vi "Interpreter.vi"(0 "string":string) -> (7 "RwZ":sgl[](array[numeric]), 8 "Yaw":sgl[](array[numeric]), 9 "RwY":sgl[](array[numeric]), 10 "Pitch":sgl[](array[numeric]), 11 "RwX":sgl[](array[numeric]), 12 "GyroX":sgl[](array[numeric]), 13 "AccZ":sgl[](array[numeric]), 14 "Roll":sgl[](array[numeric]), 15 "GyroY":sgl[](array[numeric]), 16 "Acc X":sgl[](array[numeric]), 17 "GyroZ":sgl[](array[numeric]), 18 "AccY":sgl[](array[numeric]))   [LabVIEW 2020]
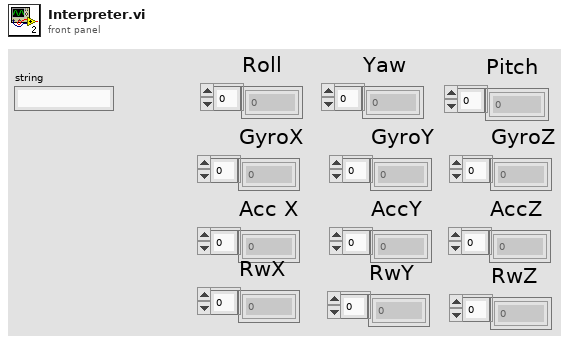
[diagram p1: front panel]
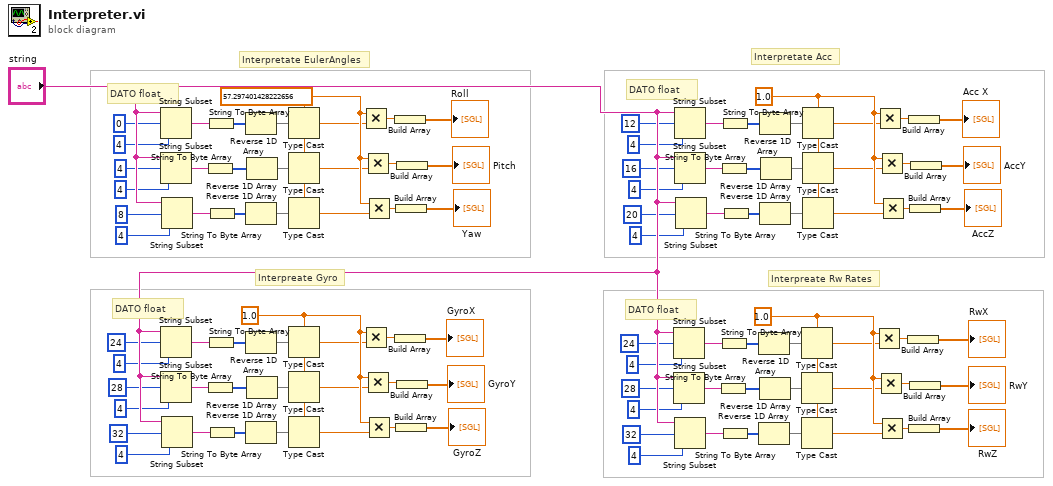
[diagram p0: block diagram]
diagram:
  w91 = sgl 1.0
  w69 = sgl 1.0
  w47 = sgl 1.0
  w22 = sgl 57.2974
  # "Interpreate Rw Rates"
  # "DATO float"
  # "Interpreate Gyro"
  # "Interpretate Acc"
  # "Interpretate EulerAngles"
  # "DATO float"
  # "DATO float"
  # "DATO float"
  n1 = String Subset(string="string", offset (0)=0, length (rest)=4 ("length (rest)")) -> (substring=w7:string)
  n2 = String Subset(string="string", offset (0)=4, length (rest)=4 ("length (rest)")) -> (substring=w8:string)
  n3 = String Subset(string="string", offset (0)=24, length (rest)=4 ("length (rest)")) -> (substring=w54:string)
  n4 = String Subset(string="string", offset (0)=28, length (rest)=4 ("length (rest)")) -> (substring=w55:string)
  n5 = String Subset(string="string", offset (0)=8, length (rest)=4 ("length (rest)")) -> (substring=w9:string)
  n6 = String Subset(string="string", offset (0)=32, length (rest)=4 ("length (rest)")) -> (substring=w56:string)
  n7 = String To Byte Array(string=w8) -> (unsigned byte array=w14:u8[])
  n8 = String To Byte Array(string=w55) -> (unsigned byte array=w61:u8[])
  n9 = String To Byte Array(string=w7) -> (unsigned byte array=w10:u8[])
  n10 = String To Byte Array(string=w54) -> (unsigned byte array=w57:u8[])
  n11 = String To Byte Array(string=w9) -> (unsigned byte array=w15:u8[])
  n12 = String To Byte Array(string=w56) -> (unsigned byte array=w62:u8[])
  n13 = Reverse 1D Array(array=w10) -> (reversed array=w11:u8[])
  n14 = Reverse 1D Array(array=w15) -> (reversed array=w13:u8[])
  n15 = Reverse 1D Array(array=w57) -> (reversed array=w58:u8[])
  n16 = Reverse 1D Array(array=w62) -> (reversed array=w60:u8[])
  n17 = Reverse 1D Array(array=w14) -> (reversed array=w12:u8[])
  n18 = Reverse 1D Array(array=w61) -> (reversed array=w59:u8[])
  n19 = Type Cast(type=w22, x=w11) -> (*(type *) &x=w17:sgl)
  n20 = Type Cast(type=w22, x=w12) -> (*(type *) &x=w18:sgl)
  n21 = Type Cast(type=w22, x=w13) -> (*(type *) &x=w19:sgl)
  n22 = Type Cast(type=w69, x=w58) -> (*(type *) &x=w64:sgl)
  n23 = Type Cast(type=w69, x=w59) -> (*(type *) &x=w65:sgl)
  n24 = Type Cast(type=w69, x=w60) -> (*(type *) &x=w66:sgl)
  n25 = Multiply(x=w22, y=w17) -> (x*y=w16:sgl)
  n26 = Multiply(x=w69, y=w64) -> (x*y=w63:sgl)
  n27 = Multiply(x=w22, y=w18) -> (x*y=w20:sgl)
  n28 = Multiply(x=w69, y=w65) -> (x*y=w67:sgl)
  n29 = Multiply(x=w22, y=w19) -> (x*y=w21:sgl)
  n30 = Multiply(x=w69, y=w66) -> (x*y=w68:sgl)
  n31 = Build Array(w16) -> (→"Roll":sgl[])
  n32 = Build Array(w63) -> (→"GyroX":sgl[])
  n33 = Build Array(w21) -> (→"Yaw":sgl[])
  n34 = Build Array(w68) -> (→"GyroZ":sgl[])
  n35 = Build Array(w20) -> (→"Pitch":sgl[])
  n36 = Build Array(w67) -> (→"GyroY":sgl[])
  n37 = String Subset(string="string", offset (0)=24, length (rest)=4 ("length (rest)")) -> (substring=w76:string)
  n38 = String Subset(string="string", offset (0)=28, length (rest)=4 ("length (rest)")) -> (substring=w77:string)
  n39 = String Subset(string="string", offset (0)=12, length (rest)=4 ("length (rest)")) -> (substring=w32:string)
  n40 = String Subset(string="string", offset (0)=16, length (rest)=4 ("length (rest)")) -> (substring=w33:string)
  n41 = String Subset(string="string", offset (0)=32, length (rest)=4 ("length (rest)")) -> (substring=w78:string)
  n42 = String Subset(string="string", offset (0)=20, length (rest)=4 ("length (rest)")) -> (substring=w34:string)
  n43 = String To Byte Array(string=w77) -> (unsigned byte array=w83:u8[])
  n44 = String To Byte Array(string=w33) -> (unsigned byte array=w39:u8[])
  n45 = String To Byte Array(string=w76) -> (unsigned byte array=w79:u8[])
  n46 = String To Byte Array(string=w32) -> (unsigned byte array=w35:u8[])
  n47 = String To Byte Array(string=w78) -> (unsigned byte array=w84:u8[])
  n48 = String To Byte Array(string=w34) -> (unsigned byte array=w40:u8[])
  n49 = Reverse 1D Array(array=w79) -> (reversed array=w80:u8[])
  n50 = Reverse 1D Array(array=w84) -> (reversed array=w82:u8[])
  n51 = Reverse 1D Array(array=w35) -> (reversed array=w36:u8[])
  n52 = Reverse 1D Array(array=w40) -> (reversed array=w38:u8[])
  n53 = Reverse 1D Array(array=w83) -> (reversed array=w81:u8[])
  n54 = Reverse 1D Array(array=w39) -> (reversed array=w37:u8[])
  n55 = Type Cast(type=w91, x=w80) -> (*(type *) &x=w86:sgl)
  n56 = Type Cast(type=w91, x=w81) -> (*(type *) &x=w87:sgl)
  n57 = Type Cast(type=w91, x=w82) -> (*(type *) &x=w88:sgl)
  n58 = Type Cast(type=w47, x=w36) -> (*(type *) &x=w42:sgl)
  n59 = Type Cast(type=w47, x=w37) -> (*(type *) &x=w43:sgl)
  n60 = Type Cast(type=w47, x=w38) -> (*(type *) &x=w44:sgl)
  n61 = Multiply(x=w91, y=w86) -> (x*y=w85:sgl)
  n62 = Multiply(x=w47, y=w42) -> (x*y=w41:sgl)
  n63 = Multiply(x=w91, y=w87) -> (x*y=w89:sgl)
  n64 = Multiply(x=w47, y=w43) -> (x*y=w45:sgl)
  n65 = Multiply(x=w91, y=w88) -> (x*y=w90:sgl)
  n66 = Multiply(x=w47, y=w44) -> (x*y=w46:sgl)
  n67 = Build Array(w85) -> (→"RwX":sgl[])
  n68 = Build Array(w41) -> (→"Acc X":sgl[])
  n69 = Build Array(w90) -> (→"RwZ":sgl[])
  n70 = Build Array(w46) -> (→"AccZ":sgl[])
  n71 = Build Array(w89) -> (→"RwY":sgl[])
  n72 = Build Array(w45) -> (→"AccY":sgl[])
